vi "Identify Tag Type.vi"(8 "Error In":errorcluster, 11 "Lexer In":refnum<class "Lexer.lvclass">) -> (0 "Error Out":errorcluster, 3 "Lexer Out":refnum<class "Lexer.lvclass">)   [LabVIEW 2018, in "Toolkit.lvlib" / "Lexer.lvclass"]
uses:
  Lexer.lvclass
  Lexer.lvclass/Lexer.ctl
  States.ctl
  Tag Types.ctl
  Is Close Delimiter.vi
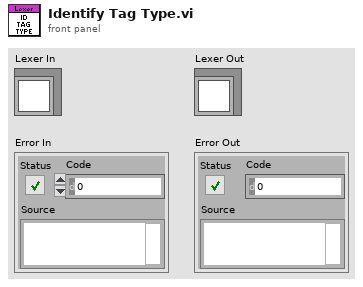
[diagram p1: front panel]
types:
  T1 = typedef "Toolkit.lvlib/Lexer.lvclass/States.ctl" = enum16{"Text", "Open Delimiter", "Tag Type", "Tag Key", "Close Delimiter"}
  T2 = typedef "Toolkit.lvlib/Lexer.lvclass/Tag Types.ctl" = enum16{"Escaped Variable", "{} Unescaped Variable", "& Unescaped Variable", "Begin Section", "Inverted Section", "End Section", "Comment", "Partial", "Set Delimiter"}
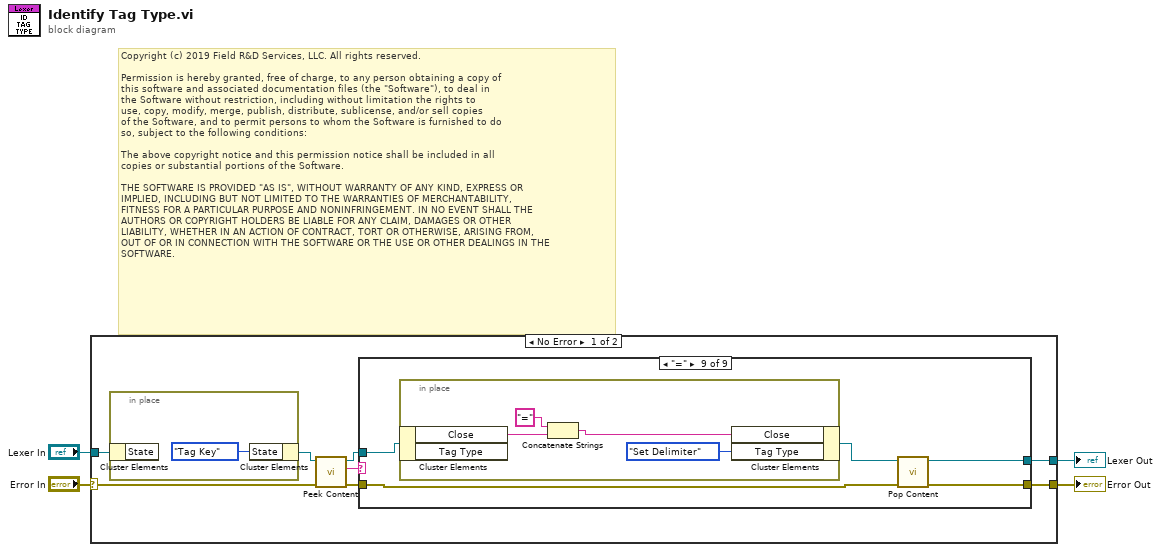
[diagram p0: block diagram]
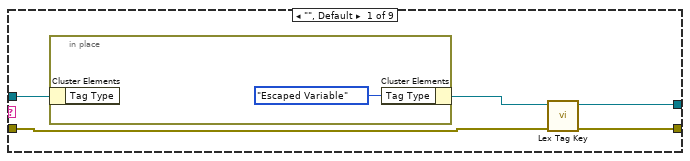
[diagram p2: hidden frame]
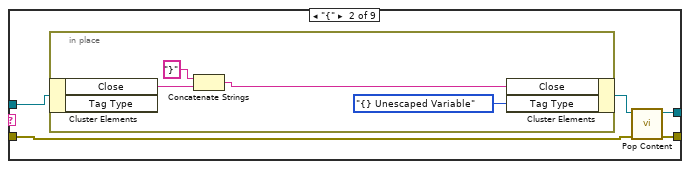
[diagram p3: hidden frame]
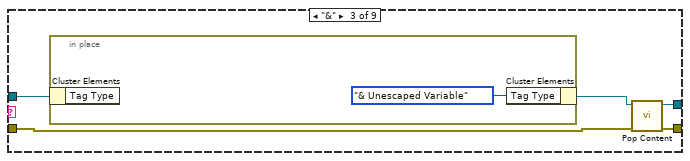
[diagram p4: hidden frame]
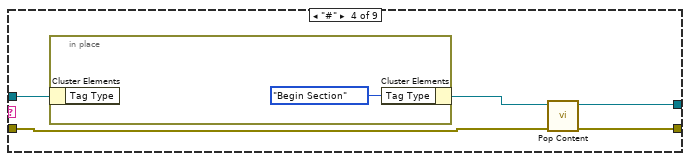
[diagram p5: hidden frame]
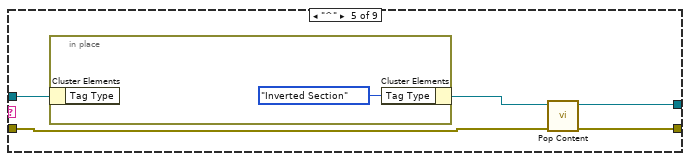
[diagram p6: hidden frame]
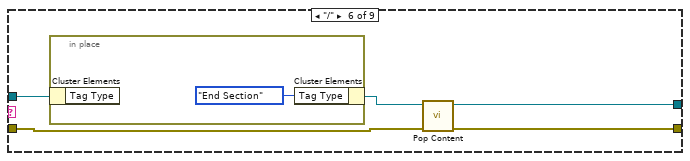
[diagram p7: hidden frame]
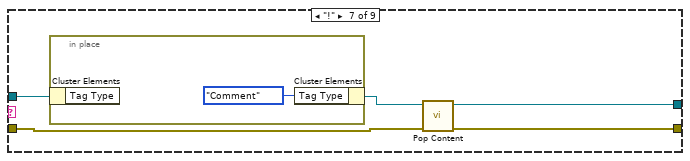
[diagram p8: hidden frame]
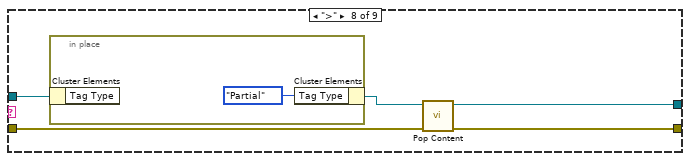
[diagram p9: hidden frame]
diagram:
  # "Copyright (c) 2019 Field R&D Services, LLC. All rights reserved.\n\nPermission is hereby granted, free of charge, to any person obtaining a copy of\nthis software and associated documentation files (the \"Software\"), to deal in\nthe Software without restriction, including without limitation the rights to\nuse, copy, modify, merge, publish, distribute, sublicense, and/or sell copies\nof the Software, and to permit persons to whom the Software is furnished to do\nso, subject to the following conditions:\n\nThe above copyright notice and this permission notice shall be included in all\ncopies or substantial portions of the Software.\n\nTHE SOFTWARE IS PROVIDED \"AS IS\", WITHOUT WARRANTY OF ANY KIND, EXPRESS OR\nIMPLIED, INCLUDING BUT NOT LIMITED TO THE WARRANTIES OF MERCHANTABILITY,\nFITNESS FOR A PARTICULAR PURPOSE AND NONINFRINGEMENT. IN NO EVENT SHALL THE\nAUTHORS OR COPYRIGHT HOLDERS BE LIABLE FOR ANY CLAIM, DAMAGES OR OTHER\nLIABILITY, WHETHER IN AN ACTION OF CONTRACT, TORT OR OTHERWISE, ARISING FROM,\nOUT OF OR IN CONNECTION WITH THE SOFTWARE OR THE USE OR OTHER DEALINGS IN THE\nSOFTWARE."
  n1 = case shown="No Error" "Error In" {
    selector: "Error In" -> [w12 w75]
    tunnel: "Lexer In" -> [w6 w74]
    tunnel: [w9 w74] -> w3
    tunnel: [w7 w75] -> w1
    frame No Error {
      n2 = in-place {
        n3 = in-place-cluster #1(w6) -> ()  [unwired: 1 out]
        n4 = in-place-cluster #1("State"=States."Tag Key") -> (w5:refnum<class "Lexer.lvclass">)
      }
      n5 = call "Peek Content.vi"("Error In"=w12, "Lexer In"=w5) -> ("Error Out"=w8:errorcluster, "Character"=w11:string, "Lexer Out"=w10:refnum<class "Lexer.lvclass">)  [unwired: 7 in]
      n6 = case shown="\"=\"" w11 {
        tunnel: w10 -> [w18 w24 w33 w39 w45 w51 w57 w63 w69]
        tunnel: [w14 w22 w31 w37 w43 w49 w55 w61 w67] -> w9
        tunnel: w8 -> [w16 w21 w30 w36 w42 w48 w54 w60 w66]
        tunnel: [w15 w20 w29 w35 w41 w47 w53 w59 w65] -> w7
        frame "", Default {
          n7 = in-place {
            n8 = in-place-cluster #2(w18) -> ()  [unwired: 1 out]
            n9 = in-place-cluster #2("Tag Type"=Tag_Types."Escaped Variable" ("Type")) -> (w17:refnum<class "Lexer.lvclass">)
          }
          n10 = call "Lex Tag Key.vi"("Error In"=w16, "Lexer In"=w17) -> ("Error Out"=w15:errorcluster, "Lexer Out"=w14:refnum<class "Lexer.lvclass">)  [unwired: 8 in]
        }
        frame "{" {
          n11 = in-place {
            n12 = in-place-cluster #3(w24) -> ("Close"=w27:string)  [unwired: 1 out]
            n13 = Concatenate Strings("}", w27) -> (w26:string)
            n14 = in-place-cluster #3("Close"=w26, "Tag Type"=Tag_Types."{} Unescaped Variable" ("Type")) -> (w23:refnum<class "Lexer.lvclass">)
          }
          n15 = call "Pop Content.vi"("Error In"=w21, "Lexer In"=w23) -> ("Error Out"=w20:errorcluster, "Lexer Out"=w22:refnum<class "Lexer.lvclass">)  [unwired: 8 in]
        }
        frame "&" {
          n16 = in-place {
            n17 = in-place-cluster #4(w33) -> ()  [unwired: 1 out]
            n18 = in-place-cluster #4("Tag Type"=Tag_Types."& Unescaped Variable") -> (w32:refnum<class "Lexer.lvclass">)
          }
          n19 = call "Pop Content.vi"("Error In"=w30, "Lexer In"=w32) -> ("Error Out"=w29:errorcluster, "Lexer Out"=w31:refnum<class "Lexer.lvclass">)  [unwired: 8 in]
        }
        frame "#" {
          n20 = in-place {
            n21 = in-place-cluster #5(w39) -> ()  [unwired: 1 out]
            n22 = in-place-cluster #5("Tag Type"=Tag_Types."Begin Section") -> (w38:refnum<class "Lexer.lvclass">)
          }
          n23 = call "Pop Content.vi"("Error In"=w36, "Lexer In"=w38) -> ("Error Out"=w35:errorcluster, "Lexer Out"=w37:refnum<class "Lexer.lvclass">)  [unwired: 8 in]
        }
        frame "^" {
          n24 = in-place {
            n25 = in-place-cluster #6(w45) -> ()  [unwired: 1 out]
            n26 = in-place-cluster #6("Tag Type"=Tag_Types."Inverted Section" ("Type")) -> (w44:refnum<class "Lexer.lvclass">)
          }
          n27 = call "Pop Content.vi"("Error In"=w42, "Lexer In"=w44) -> ("Error Out"=w41:errorcluster, "Lexer Out"=w43:refnum<class "Lexer.lvclass">)  [unwired: 8 in]
        }
        frame "/" {
          n28 = in-place {
            n29 = in-place-cluster #7(w51) -> ()  [unwired: 1 out]
            n30 = in-place-cluster #7("Tag Type"=Tag_Types."End Section" ("Type")) -> (w50:refnum<class "Lexer.lvclass">)
          }
          n31 = call "Pop Content.vi"("Error In"=w48, "Lexer In"=w50) -> ("Error Out"=w47:errorcluster, "Lexer Out"=w49:refnum<class "Lexer.lvclass">)  [unwired: 8 in]
        }
        frame "!" {
          n32 = in-place {
            n33 = in-place-cluster #8(w57) -> ()  [unwired: 1 out]
            n34 = in-place-cluster #8("Tag Type"=Tag_Types."Comment" ("Type")) -> (w56:refnum<class "Lexer.lvclass">)
          }
          n35 = call "Pop Content.vi"("Error In"=w54, "Lexer In"=w56) -> ("Error Out"=w53:errorcluster, "Lexer Out"=w55:refnum<class "Lexer.lvclass">)  [unwired: 8 in]
        }
        frame ">" {
          n36 = in-place {
            n37 = in-place-cluster #9(w63) -> ()  [unwired: 1 out]
            n38 = in-place-cluster #9("Tag Type"=Tag_Types."Partial" ("Type")) -> (w62:refnum<class "Lexer.lvclass">)
          }
          n39 = call "Pop Content.vi"("Error In"=w60, "Lexer In"=w62) -> ("Error Out"=w59:errorcluster, "Lexer Out"=w61:refnum<class "Lexer.lvclass">)  [unwired: 8 in]
        }
        frame "=" {
          n40 = in-place {
            n41 = in-place-cluster #10(w69) -> ("Close"=w72:string)  [unwired: 1 out]
            n42 = Concatenate Strings("=", w72) -> (w71:string)
            n43 = in-place-cluster #10("Close"=w71, "Tag Type"=Tag_Types."Set Delimiter" ("Type")) -> (w68:refnum<class "Lexer.lvclass">)
          }
          n44 = call "Pop Content.vi"("Error In"=w66, "Lexer In"=w68) -> ("Error Out"=w65:errorcluster, "Lexer Out"=w67:refnum<class "Lexer.lvclass">)  [unwired: 8 in]
        }
      }
    }
    frame Error {
    }
  }
  "Lexer Out" <- w3
  "Error Out" <- w1
